vi "shutdown.vi"(8 "error in":errorcluster, 11 "Target Runtime in":refnum<class "PL_Target RIO Runtime.lvclass">) -> (0 "error out":errorcluster)   [LabVIEW 2013, in "PL_Target RIO Runtime.lvclass"]
doc: "Performs any shutdown operations necessary to close any references initialized by the target. This should be called last after shutting down all engines and modules used by the target."
uses:
  PL_Target RIO Runtime.lvclass
  target runtime/PL_Target Runtime.lvclass
  <vilib>/NI/Tag Bus Module Framework/FPGA manager/methods.ctl
  <vilib>/NI/Tag Bus Module Framework/FPGA manager/FPGA manager.lvlib
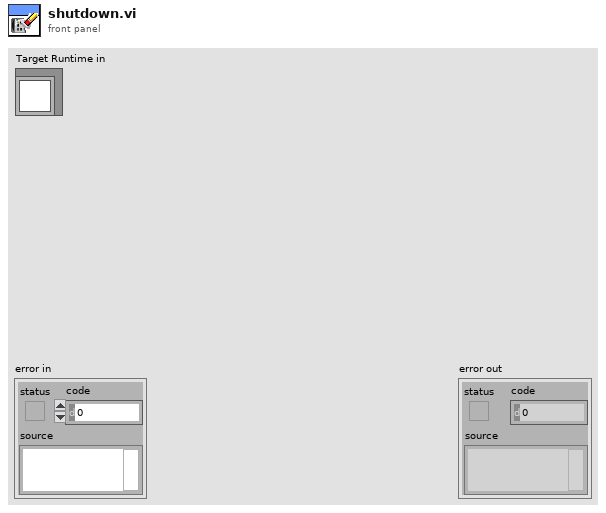
[diagram p1: front panel]
types:
  T1 = typedef "FPGA manager.lvlib/methods.ctl" = enum16{"initialize bitfile", "cache bitfile", "locate bitfile", "close bitfile", "clear manager"}
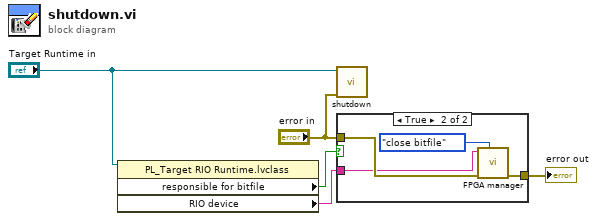
[diagram p0: block diagram]
diagram:
  n1 = property class="PL_Target RIO Runtime.lvclass"(reference="Target Runtime in") -> ("responsible for bitfile"=w2:bool, "RIO device"=w1:string)  [unwired: 1 in, 2 out]
  n2 = call-parent "shutdown.vi"("error in"="error in", "Target Runtime in"="Target Runtime in") -> ()  [unwired: 9 in, 1 out]
  n3 = case shown="True" w2 {
    tunnel: "error in" -> [w6 w9]
    tunnel: [w6 w8] -> w4
    tunnel: w1 -> [_ w7]
    frame False {
    }
    frame True {
      n4 = call <vilib>:"FPGA manager.vi"("action"=methods."close bitfile", "error in"=w9, "RIO resource"=w7) -> ("error out"=w8:errorcluster)  [unwired: 6 in, 2 out]
    }
  }
  "error out" <- w4
